vi "WriteData.vi"(8 "error in (no error)":errorcluster, 9 "t0":timestamp, 10 "data value":dbl[][](array[numeric]), 11 "Wvfrm_ref":T1={"t0"=timestamp(0 s since 1904-01-01), "dt"=1.0, "attributes"=variant, "Y_ref"=refnum} {"dt" format="%0.6f"; "t0" format="%<%X\n%x>T"}) -> (0 "error out":errorcluster, 2 "data value":dbl[][](array[numeric]), 3 "Wvfrm_ref":T1={"t0"=timestamp(0 s since 1904-01-01), "dt"=1.0, "attributes"=variant, "Y_ref"=refnum} {"dt" format="%0.6f"; "t0" format="%<%X\n%x>T"})   [LabVIEW 2018, in "AnalysisPlugins.lvlib" / "FitterBase.lvclass"]
uses:
  FitterBase.lvclass
  Typedefs/Wvfrm_ref.ctl
  Digitizer/DigitizerPlugins/DigitizerBaseClass/Typedefs/WfrmAttributes.ctl
  Digitizer/DigitizerPlugins/DigitizerBaseClass/DigitizerBase.lvclass
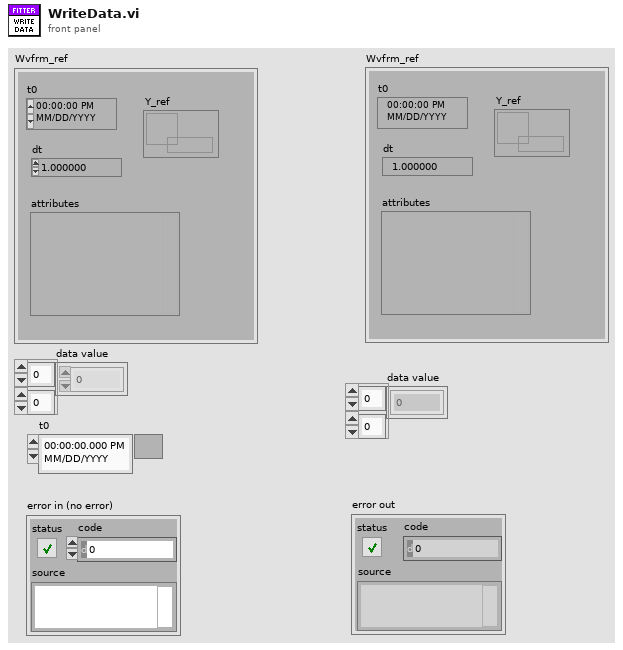
[diagram p1: front panel]
types:
  T1 = typedef "AnalysisPlugins.lvlib/FitterBase.lvclass/Wvfrm_ref.ctl" = cluster{"t0":timestamp, "dt":dbl, "attributes":variant, "Y_ref":refnum<data-value>}
  T2 = typedef "DigitizerPlugins.lvlib/DigitizerBase.lvclass/WfrmAttributes.ctl" = cluster{"XOffset":dbl, "ActualPts":i64, "FirstValid":i64}
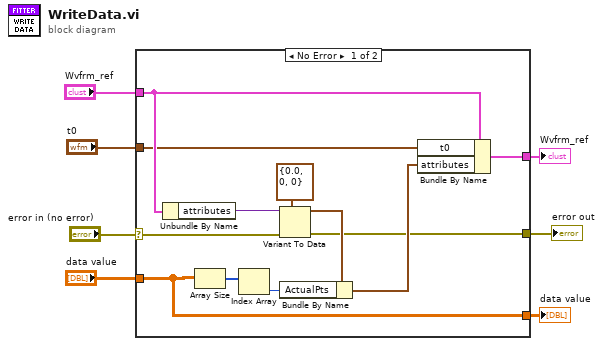
[diagram p0: block diagram]
diagram:
  n1 = case shown="No Error" "error in (no error)" {
    selector: "error in (no error)" -> [w14 w21]
    tunnel: "Wvfrm_ref" -> [w19 w22]
    tunnel: "data value" -> [w8 w20]
    tunnel: "t0" -> [w12 _]
    tunnel: [w10 w22] -> w3
    tunnel: [w9 w21] -> w2
    tunnel: [w8 w20] -> w1
    frame No Error {
      n2 = Unbundle By Name(w19) -> ("attributes"=w15:variant)
      n3 = Array Size(array=w8) -> (size(s)=w18:i32[])
      n4 = Index Array(array=w18) -> (element=w17:i32)  [unwired: 1 in]
      n5 = Variant To Data(error in=w14, type=T2 {"XOffset"=0.0, "ActualPts"=0, "FirstValid"=0} ("Attributes"), Variant=w15) -> (data=w13:T2, error out=w9:errorcluster)
      n6 = Bundle By Name(cluster=w13, "ActualPts"=w17) -> (w11:T2)
      n7 = Bundle By Name(cluster=w19, "t0"=w12, "attributes"=w11) -> (w10:T1)
    }
    frame Error {
    }
  }
  "Wvfrm_ref" <- w3
  "error out" <- w2
  "data value" <- w1
